vi "test verify value - alternate v2.vi"() -> ()   [LabVIEW 2017]
uses:
  <vilib>/TELLC/Misc Utilities/AB Settings--cluster.ctl
panel:
  in  "Mode":enum16{"Band", "UpperLimit", "LowerLimit"}(ring)
  out "InRange?":bool
  out "Fault?":bool
  out "Warning?":bool
  in  "Settings":T1={"AnalogBand Enable"=FALSE, "Fault(%)"=1.0, "Warning(%)"=5.0, "Stabilization time (ms)"=2000} {"Fault(%)" format="%#_g%%"; "Warning(%)" format="%#_g%%"}
  in  "Actual Value":dbl
  in  "Set Point":dbl
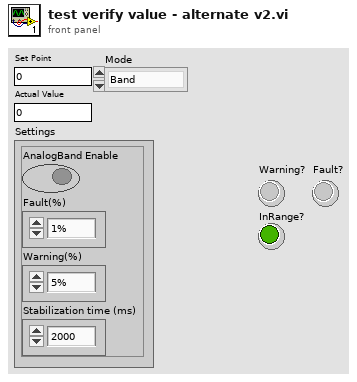
[diagram p1: front panel]
types:
  T1 = typedef "AB Settings--cluster.ctl" = cluster{"AnalogBand Enable":bool, "Fault(%)":dbl, "Warning(%)":dbl, "Stabilization time (ms)":u32}
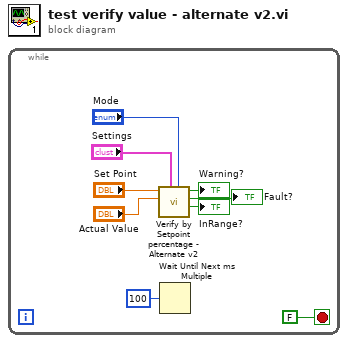
[diagram p0: block diagram]
diagram:
  n1 = while {
    stop <- FALSE stop-if-true
    n2 = call "Verify by Setpoint percentage - Alternate v2.vi"("Mode"="Mode", "Settings"="Settings", "Actual Value"="Actual Value", "Set Point"="Set Point") -> ("InRange?"=→"InRange?":bool, "Fault?"=→"Fault?":bool, "Warning?"=→"Warning?":bool)  [unwired: 5 in]
    n3 = Wait Until Next ms Multiple(millisecond multiple=u32 100) -> ()  [unwired: 1 out]
  }
